vi "helper--Set Control Tags.vi"() -> ()   [LabVIEW 2024]
doc: "set the control tags correctly for all of the button types in the directory\n\n<b>Code Developed By:</b>\nTechnology Service Corporation\n1983 S Liberty Drive\nBloomington, IN 47403\nPhone: 812 558-7100\nwww.tsc.com/atcs\n\nDeveloper:\nDaniel Coons"
panel:
  in  "Tag Name":string="button-type"
  out "error out":errorcluster
  # "UI Theme:\nN/A\nPrimary\nSecondary\nTertiary\nNo Change"
  # "Control Types:\noutline--icon--rounded\noutline--text--rounded\nnooutline--icon--rounded\nnooutline--text--rounded\ntonal--icon--rounded\ntonal--text--rounded\nfilled--icon--rounded\nfilled--text--rounded"
  # "Control Types:\noutline--icon--rectangular\noutline--text--rectangular\nnooutline--icon--rectangular\nnooutline--text--rectangular\ntonal--icon--rectangular\ntonal--text--rectangular\nfilled--icon--rectangular\nfilled--text--rectangular"
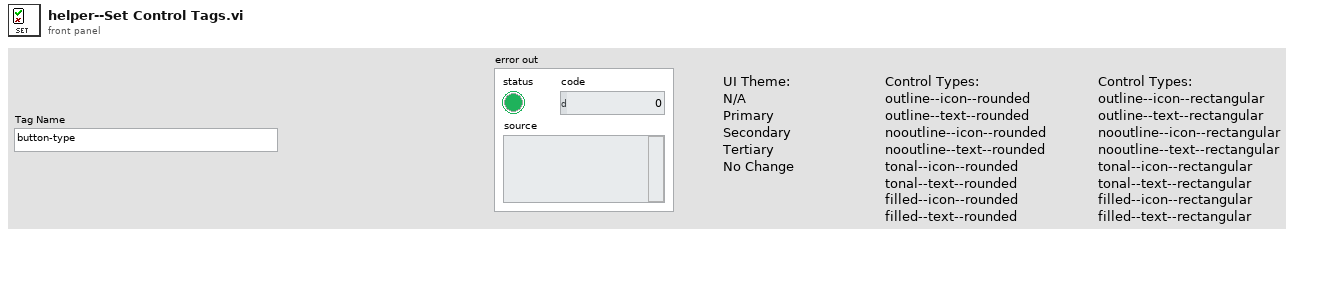
[diagram p1: front panel]
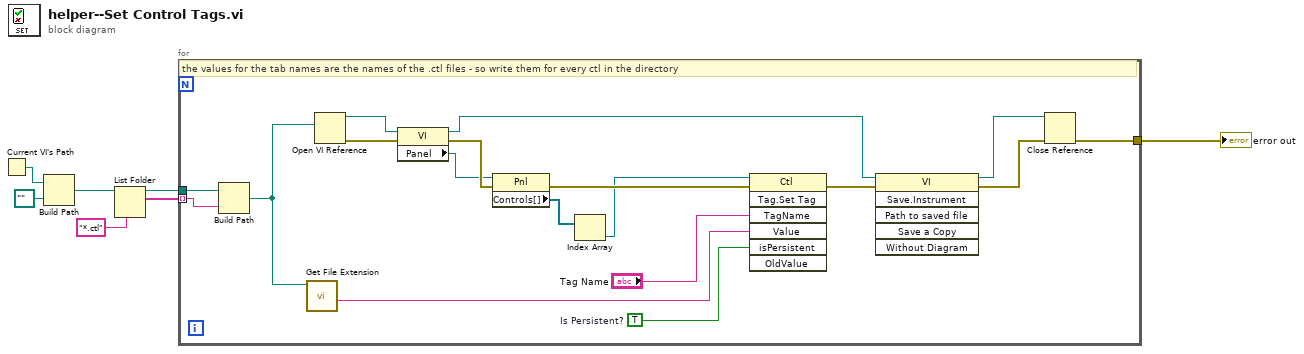
[diagram p0: block diagram]
diagram:
  n1 = Current VI's Path() -> (path=w6:path)
  n2 = Build Path(base path=w6, name or relative path=path "..") -> (appended path=w4:path)
  n3 = List Folder(path=w4, pattern="*.ctl") -> (path out=w2:path, filenames=w1:string[])  [unwired: 2 in, 2 out]
  n4 = for {
    tunnel: [w19] -> w7
    tunnel: w2 -> [w14]
    tunnel: w1 -> [w13] mode=indexing
    w16 = TRUE  # Is Persistent?
    # "the values for the tab names are the names of the .ctl files - so write them for every ctl in the directory"
    n5 = Build Path(base path=w14, name or relative path=w13) -> (appended path=w12:path)
    n6 = call <vilib>:"Get File Extension.vi"("file"=w12) -> ("filename without extension"=w11:string)  [unwired: 6 in, 4 out]
    n7 = Open VI Reference(vi path=w12) -> (vi reference=w23:refnum<vi>, error out=w25:errorcluster)  [unwired: 5 in]
    n8 = property class="VI"(reference=w23, error in=w25) -> (reference out=w9:refnum<vi>, error out=w24:errorcluster, "Panel"=w21:refnum<vi>)
    n9 = property class="Pnl"(reference=w21, error in=w24) -> (error out=w22:errorcluster, "Controls[]"=w20:refnum<vi>[])  [unwired: 1 out]
    n10 = Index Array(array=w20) -> (element=w17:refnum<vi>)  [unwired: 1 in]
    n11 = invoke class="Ctl" method="Tag.Set Tag"(reference=w17, error in=w22, "TagName"="Tag Name", "Value"=w11, "isPersistent"=w16) -> (error out=w18:errorcluster)  [unwired: 2 in, 6 out]
    n12 = invoke class="VI" method="Save.Instrument"(reference=w9, error in=w18) -> (reference out=w8:refnum<vi>, error out=w10:errorcluster)  [unwired: 4 in, 4 out]
    n13 = Close Reference(reference=w8, error in (no error)=w10) -> (error out=w19:errorcluster)
  }
  "error out" <- w7
